vi "data to map setting.vi"(8 "error in (no error)":errorcluster, 11 "data in":string[](array[string])) -> (0 "error out":errorcluster, 3 "<JSON>":string)   [LabVIEW 2019]
uses:
  <vilib>/JDP Science/JSONtext/support/Format JSON Array Text.vi
  <vilib>/JDP Science/JSONtext/support/Format JSON Object.vi
  <vilib>/JDP Science/JSONtext/JSONtext.lvlib
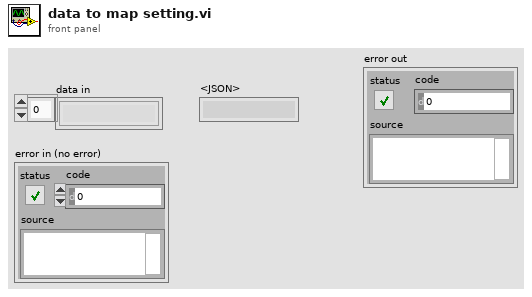
[diagram p1: front panel]
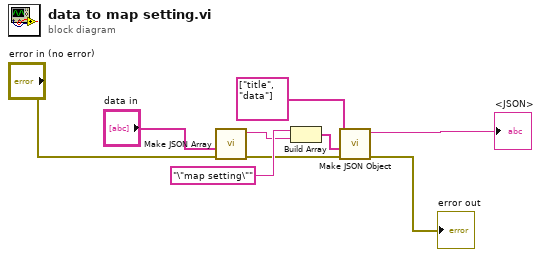
[diagram p0: block diagram]
diagram:
  n1 = call <vilib>:"Make JSON Array.vi"("error in (no error)"="error in (no error)", "JSON Elements"="data in") -> ("error out"=w4:errorcluster, "<JSON>"=w8:string)  [unwired: 8 in]
  n2 = Build Array("\"map setting\"" ("element"), w8) -> (w5:string[])
  n3 = call <vilib>:"Make JSON Object.vi"("error in (no error)"=w4, "JSON Items"=w5, "Item Names"=string[] ["title", "data"]) -> ("error out"=→"error out":errorcluster, "<JSON>"=→"<JSON>":string)  [unwired: 7 in]
